vi "Add Attachment.vi"(8 "error in (no error)":errorcluster caption="错误输入（无错误）", 10 "Attachment File":path, 11 "Email In":refnum<class "Email.lvclass"> caption="DNL_LabVIEW Object in") -> (0 "error out":errorcluster caption="错误输出", 3 "Email Out":refnum<class "Email.lvclass"> caption="DNL_LabVIEW Object out")   [LabVIEW 2012, in "Email.lvclass"]
uses:
  Email.lvclass
  Email.lvclass/Email.ctl
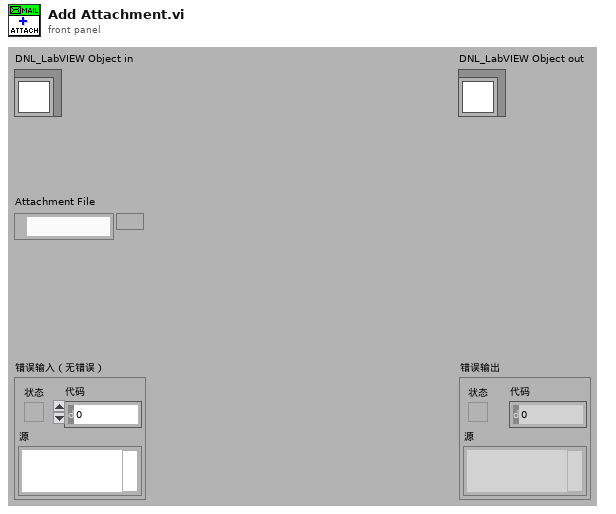
[diagram p1: front panel]
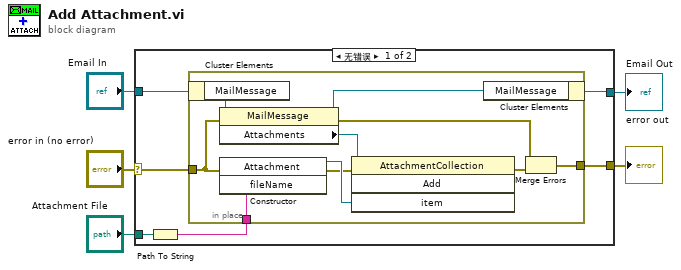
[diagram p0: block diagram]
diagram:
  n1 = case shown="无错误" "error in (no error)" {
    selector: "error in (no error)" -> [w8 w23]
    tunnel: [w7 w23] -> w4
    tunnel: [w6 w22] -> w2
    tunnel: "Email In" -> [w11 w22]
    tunnel: "Attachment File" -> [w10 _]
    frame No Error {
      n2 = Path To String(path=w10) -> (string=w9:string)
      n3 = in-place {
        in-place-border: w9 -> [w19]
        in-place-border: w8 -> [w17]
        in-place-border: [w12] -> w7
        n4 = in-place-cluster #1(w11) -> ("MailMessage"=w21:refnum<k24>)
        n5 = property class="MailMessage"(reference=w21, error in=w17) -> (reference out=w13:refnum<k24>, error out=w15:errorcluster, "Attachments"=w20:refnum<k24>)
        n6 = constructor class="Attachment"(error in=w17, "fileName"=w19) -> (reference out=w18:refnum<k24>, error out=w16:errorcluster)  [unwired: 2 in, 2 out]
        n7 = invoke class="AttachmentCollection" method="Add"(reference=w20, error in=w16, "item"=w18) -> (error out=w14:errorcluster)  [unwired: 1 in, 3 out]
        n8 = in-place-cluster #1("MailMessage"=w13) -> (w6:refnum<class "Email.lvclass">)
        n9 = Merge Errors(w15, w14) -> (w12:errorcluster)
      }
    }
    frame Error {
    }
  }
  "error out" <- w4
  "Email Out" <- w2
